vi "ConfirmSerialNo.vi"(0 "Manufacturer":string, 1 "Device Type":string, 2 "Manufacturer SN":string, 3 "SCT SN":string) -> ()   [LabVIEW 2018]
panel:
  in  "OK Button":bool
  out "Device Type":string
  out "Manufacturer:":string
  out "ATLAS Serial No.:":string
  # "Database Record for this sensor"
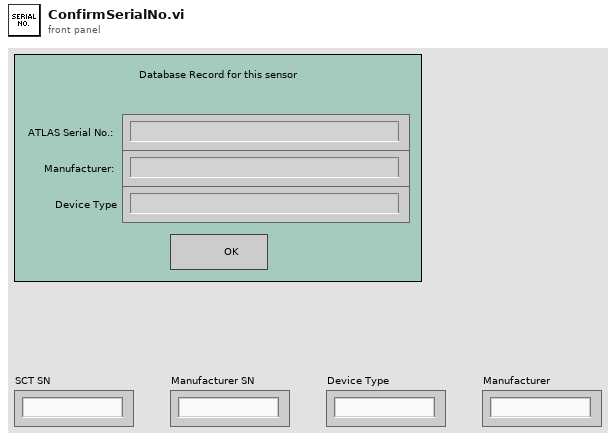
[diagram p1: front panel]
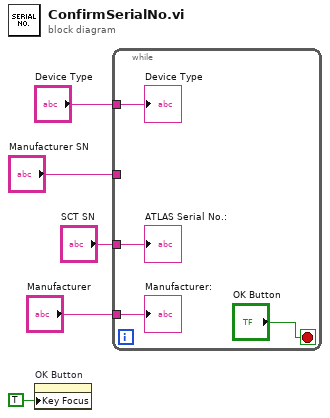
[diagram p0: block diagram]
diagram:
  n1 = property on="OK Button" class="Bool"("Key Focus"=TRUE) -> ()  [unwired: 2 in, 2 out]
  n2 = while {
    tunnel: "SCT SN" -> [w8]
    tunnel: "Manufacturer" -> [w6]
    tunnel: "Device Type" -> [w7]
    tunnel: "Manufacturer SN" -> [_]
    stop <- "OK Button" stop-if-true
    "Manufacturer:" <- w6
    "ATLAS Serial No.:" <- w8
    "Device Type" <- w7
  }
